vi "AlliGator Check Available Buffer Image.vi"(6 "Image Characteristics":T2 {"Calibration"."Y Step" format="%.2f"; "Calibration"."X Step" format="%.2f"; "Image Type" items=["Grayscale (U8)", "Grayscale (I16)", "Grayscale (SGL)", "Complex (CSG)", "RGB (U32)", "HSL (U32)", "RGB (U64)", "Grayscale (U16)"]}, 7 "Buffer Image available?":bool, 8 "error in (no error)":errorcluster, 9 "Current Gate":i32, 11 "Image Buffer":T1[](array[typedef])) -> (0 "error out":errorcluster, 1 "Same Image Type?":bool, 2 "Image Reused?":bool, 3 "Gate Image":T1)   [LabVIEW 2021, in "AlliGator Files.lvlib"]
doc: "Checks whether the buffer already contains an image structure for the new loaded gate image.\n\nIf yes, returns it. If not, creates a new image structure."
uses:
  Image/Image Characteristics.ctl
  <vilib>/vision/Image Controls.llb/IMAQ Image.ctl
  AlliGator Files.lvlib
  Image/Image.lvlib
panel:
  # "see the AlliGator License on the block diagram (Ctrl+E or Window:Show Block Diagram)"
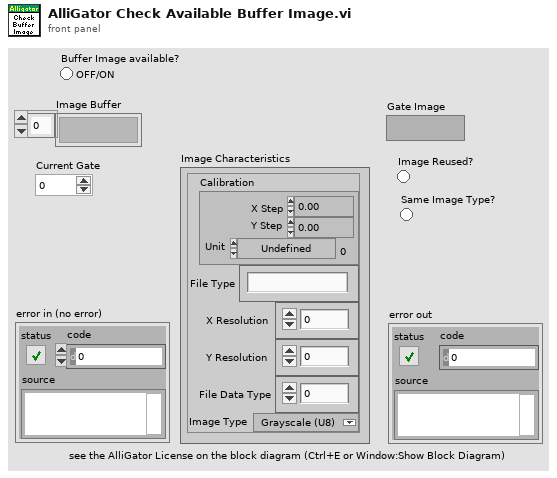
[diagram p1: front panel]
types:
  T1 = typedef "IMAQ Image.ctl" = refnum<image>
  T2 = typedef "Image.lvlib/Image Characteristics.ctl" = cluster{"Calibration":T3, "File Type":string, "X Resolution":i32, "Y Resolution":i32, "File Data Type":i32, "Image Type":T5}
  T3 = typedef "Simple Grid Descriptor" = cluster{"X Step":sgl, "Y Step":sgl, "Unit":T4}
  T4 = typedef "Image Unit" = enum32{"Undefined", "Angström", "Micrometer", "Millimeter", "Centimeter", "Meter", "Kilometer", "Microinch", "Inch", "Feet", "Nautical miles", "Standard miles", "Steps"}
  T5 = typedef "Image Type" = u32
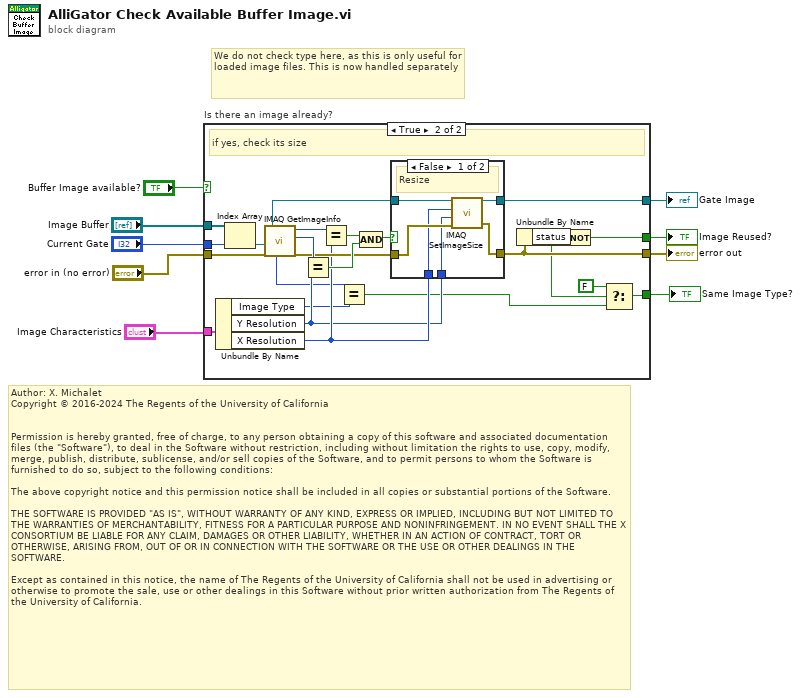
[diagram p0: block diagram]
diagram:
  # "Author: X. Michalet\nCopyright © 2016-2024 The Regents of the University of California\n \n\nPermission is hereby granted, free of charge, to any person obtaining a copy of this software and associated documentation files (the \"Software\"), to deal in the Software without restriction, including without limitation the rights to use, copy, modify, merge, publish, distribute, sublicense, and/or sell copies of the Software, and to permit persons to whom the Software is furnished to do so, subject to the following conditions:\n\nThe above copyright notice and this permission notice shall be included in all copies or substantial portions of the Software.\n\nTHE SOFTWARE IS PROVIDED \"AS IS\", WITHOUT WARRANTY OF ANY KIND, EXPRESS OR IMPLIED, INCLUDING BUT NOT LIMITED TO THE WARRANTIES OF MERCHANTABILITY, FITNESS FOR A PARTICULAR PURPOSE AND NONINFRINGEMENT. IN NO EVENT SHALL THE X CONSORTIUM BE LIABLE FOR ANY CLAIM, DAMAGES OR OTHER LIABILITY, WHETHER IN AN ACTION OF CONTRACT, TORT OR OTHERWISE, ARISING FROM, OUT OF OR IN CONNECTION WITH THE SOFTWARE OR THE USE OR OTHER DEALINGS IN THE SOFTWARE.\n\nExcept as contained in this notice, the name of The Regents of the University of California shall not be used in advertising or otherwise to promote the sale, use or other dealings in this Software without prior written authorization from The Regents of the University of California."
  # "We do not check type here, as this is only useful for loaded image files. This is now handled separately"
  n1 = case "Is there an image already?" shown="True" "Buffer Image available?" {
    tunnel: "Image Buffer" -> [_ w32]
    tunnel: "Current Gate" -> [_ w31]
    tunnel: "error in (no error)" -> [w10 w30]
    tunnel: [w10 w16] -> w4
    tunnel: [_ w24] -> w5
    tunnel: [_ w15] -> w6
    tunnel: "Image Characteristics" -> [_ w22]
    tunnel: [_ w11] -> w1
    frame False {
    }
    frame True {
      # "if yes, check its size"
      n2 = Unbundle By Name(w22) -> ("Image Type"=w17:T5, "Y Resolution"=w19:i32, "X Resolution"=w20:i32)
      n3 = Index Array(array=w32, index=w31) -> (element=w25:T1)
      n4 = call "IMAQ GetImageInfo"("error in (no error)"=w30, "Image"=w25) -> ("error out"=w21:errorcluster, "Y Resolution"=w28:i32, "X Resolution"=w29:i32, "Image Type"=w18:T5)  [unwired: 2 in, 4 out]
      n5 = Equal?(x=w28, y=w19) -> (x = y?=w26:bool)
      n6 = Equal?(x=w29, y=w20) -> (x = y?=w27:bool)
      n7 = Equal?(x=w18, y=w17) -> (x = y?=w13:bool)
      n8 = Compound Arithmetic op=AND(w27, w26) -> (w23:bool)
      n9 = case shown="False" w23 {
        tunnel: w25 -> [w38 w40]
        tunnel: [w37 w40] -> w24
        tunnel: w21 -> [w36 w39]
        tunnel: [w35 w39] -> w16
        tunnel: w20 -> [w34 _]
        tunnel: w19 -> [w33 _]
        frame False {
          # "Resize"
          n10 = call "IMAQ SetImageSize"("error in (no error)"=w36, "Y Resolution"=w33, "X Resolution"=w34, "Image"=w38) -> ("error out"=w35:errorcluster, "Image Out"=w37:T1)  [unwired: 1 in]
        }
        frame True {
          # "Keep"
        }
      }
      n11 = Unbundle By Name(w16) -> ("status"=w14:bool)
      n12 = Not(x=w14) -> (.not. x?=w15:bool)
      n13 = Select(t=FALSE, s=w14, f=w13) -> (s? t:f=w11:bool)
    }
  }
  "Image Reused?" <- w6
  "Gate Image" <- w5
  "error out" <- w4
  "Same Image Type?" <- w1
